vi "AOD.vi"() -> ()   [LabVIEW 2012]
uses:
  <vilib>/DAQmx/configure/timing.llb/DAQmx Timing (Sample Clock).vi
  <vilib>/DAQmx/configure/trigger.llb/DAQmx Start Trigger (Digital Edge).vi
  <resource>/objmgr/daqmx.rc
  <vilib>/DAQmx/configure/timing.llb/DAQmx Timing (Implicit).vi
  <vilib>/DAQmx/read.llb/DAQmx Read (Analog 1D Wfm NChan NSamp).vi
  <instrlib>/niHWS/nihws.llb/niHWS Open File Permissions ID.ctl
  <instrlib>/niHWS/nihws.llb/niHWS Write Analog WDT.vi
  <vilib>/DAQmx/read.llb/DAQmx Read (Digital 2D U32 NChan NSamp).vi
  <instrlib>/niHWS/nihws.llb/niHWS Write Digital 2D U32.vi
panel:
  in  "Channel":i32
  in  "Record":bool
  in  "Construct image":bool=TRUE
  in  "Show traces":bool
  in  "samples per ch":i32=5000
  out "PMT Waveforms":waveform(dbl)[](graph)
  out "Sync Signals":digitalwaveform(graph)
  out "Numeric":i32
  in  "stop":bool
  in  "buffer size":i32=10000000
  in  "pulse width (us)":dbl=5.0 format="%#.6f"
  in  "pixel oversampling":dbl=4.0
  in  "pixel rate":dbl=50000.0 format="%0.0f"
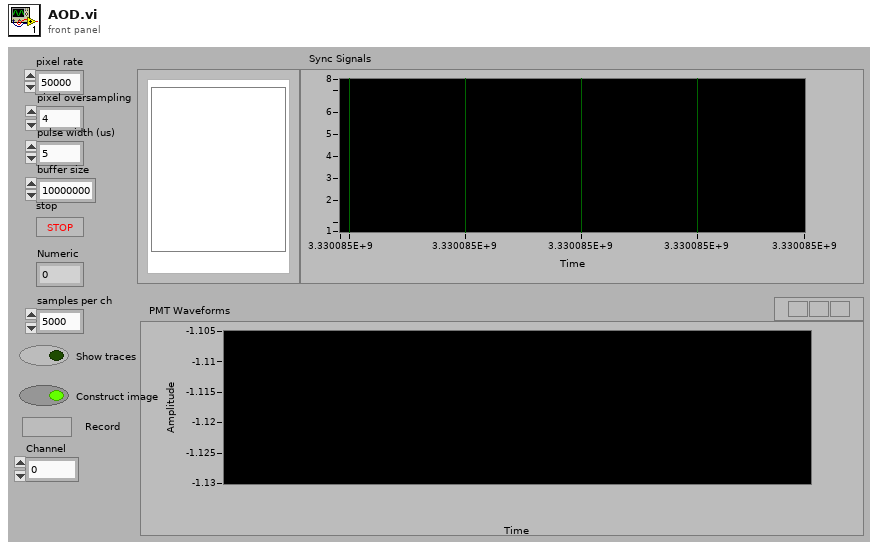
[diagram p1: front panel]
types:
  T1 = typedef "niHWS Open File Permissions ID.ctl" = enum32{"Read Only", "Read/Write Existing", "Read/Write/Create New", "Read/Write/Create New Always"}
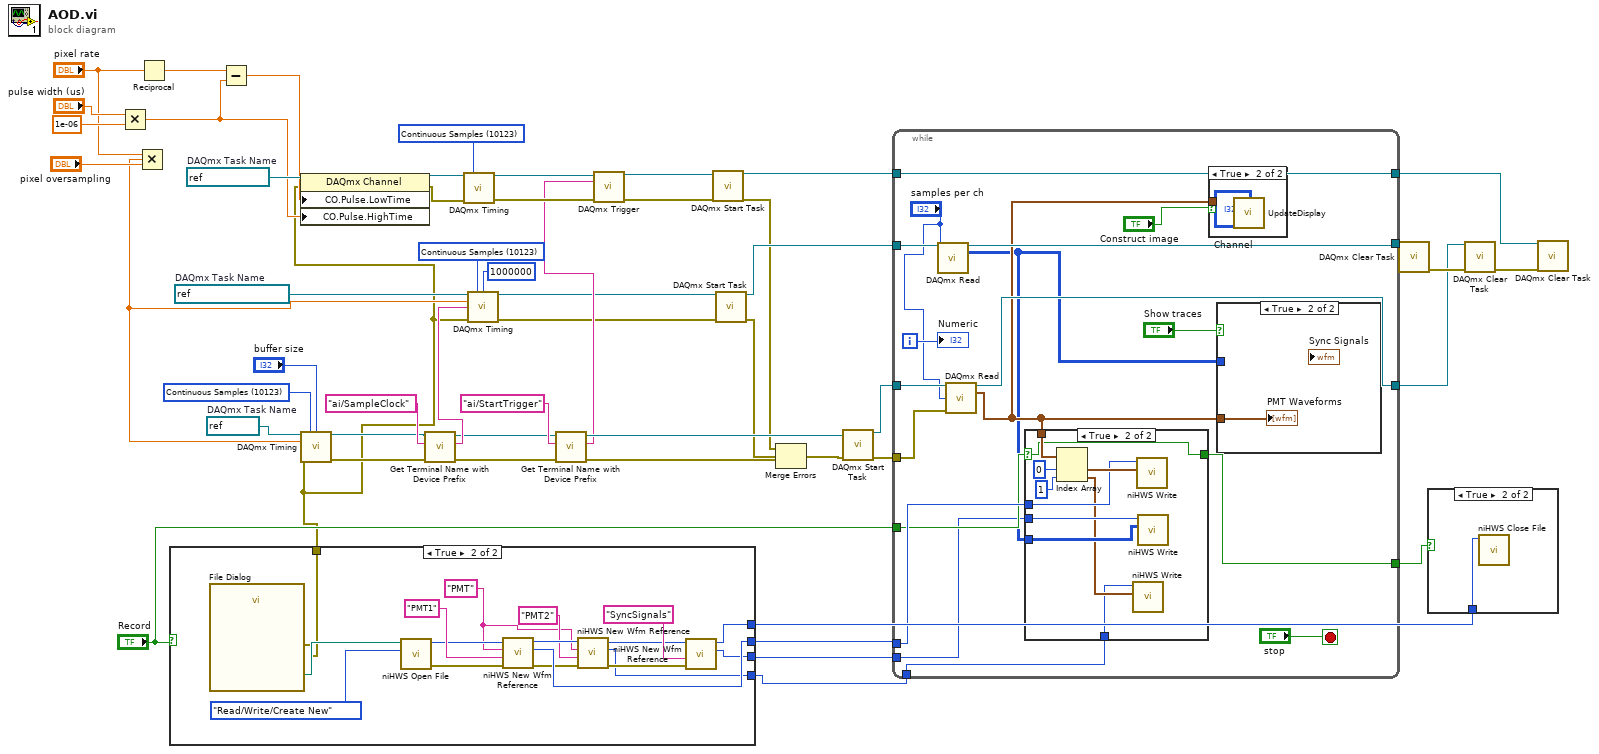
[diagram p0: block diagram]
diagram:
  w6 = 10123 items=["Finite Samples"=10178, "Continuous Samples"=10123, "Hardware Timed Single Point"=12522] ("sample mode")
  w36 = refnum<k21> "AODSyncSignals"  # DAQmx Task Name
  w42 = refnum<k21> "AODClock"  # DAQmx Task Name
  w47 = 10123 items=["Finite Samples"=10178, "Continuous Samples"=10123, "Hardware Timed Single Point"=12522] ("sample mode")
  w51 = refnum<k21> "PMT"  # DAQmx Task Name
  w53 = 10123 items=["Finite Samples"=10178, "Continuous Samples"=10123, "Hardware Timed Single Point"=12522] ("sample mode")
  n1 = Multiply(x="pulse width (us)", y=1e-06) -> (x*y=w37:dbl)
  n2 = Multiply(x="pixel rate", y="pixel oversampling") -> (x*y=w12:dbl)
  n3 = Reciprocal(x="pixel rate") -> (1/x=w39:dbl)
  n4 = case shown="True" "Record" {
    tunnel: [_ w67] -> w10
    tunnel: [_ w66] -> w8
    tunnel: [_ w63] -> w7
    tunnel: [_ w61] -> w2
    tunnel: [_ w54] -> w1
    frame False {
    }
    frame True {
      w55 = "PMT" ("group name (empty)")
      n5 = call "File Dialog"() -> ("selected path"=w62:path, "error out"=w61:errorcluster)  [unwired: 7 in, 7 out]
      n6 = call <instrlib>:"niHWS Open File.vi"("permissions (0:read only)"=niHWS_Open_File_Permissions_ID."Read/Write/Create New", "file path"=w62) -> ("error out"=w64:errorcluster, "file handle"=w68:u32)  [unwired: 1 in, 7 out]
      n7 = call <instrlib>:"niHWS New Wfm Reference.vi"("error in (no error)"=w64, "waveform name (empty)"="PMT1", "group name (empty)"=w55, "file handle in"=w68) -> ("error out"=w59:errorcluster, "waveform reference"=w67:u32, "file handle out"=w60:u32)  [unwired: 1 in, 4 out]
      n8 = call <instrlib>:"niHWS New Wfm Reference.vi"("error in (no error)"=w59, "waveform name (empty)"="PMT2", "group name (empty)"=w55, "file handle in"=w60) -> ("error out"=w58:errorcluster, "waveform reference"=w54:u32, "file handle out"=w57:u32)  [unwired: 1 in, 4 out]
      n9 = call <instrlib>:"niHWS New Wfm Reference.vi"("error in (no error)"=w58, "waveform name (empty)"="SyncSignals", "file handle in"=w57) -> ("waveform reference"=w63:u32, "file handle out"=w66:u32)  [unwired: 1 in, 6 out]
    }
  }
  n10 = Subtract(x=w39, y=w37) -> (x-y=w38:dbl)
  n11 = property class="DAQmx Channel"(reference=w42, error in=w2, "CO.Pulse.LowTime"=w38, "CO.Pulse.HighTime"=w37) -> (reference out=w40:refnum<k21>, error out=w41:errorcluster)
  n12 = call-poly <vilib>:"DAQmx Timing.vi"("task/channels in"=w51, "sample mode"=w47, "samples per channel"="buffer size", "rate"=w12, "error in"=w2) -> ("task out"=w30:refnum<k21>, "error out"=w35:errorcluster)  [unwired: 2 in, 7 out]
  n13 = call "Get Terminal Name with Device Prefix.vi"("error in (no error)"=w35, "Local Terminal Name"="ai/SampleClock", "task/channels in"=w30) -> ("error out"=w29:errorcluster, "Terminal Name with Device Prefix"=w33:tag, "task out"=w28:refnum<k21>)  [unwired: 1 in, 5 out]
  n14 = call-poly <vilib>:"DAQmx Timing.vi"("task/channels in"=w40, "sample mode"=w53, "error in"=w41) -> ("task out"=w46:refnum<k21>, "error out"=w45:errorcluster)  [unwired: 3 in, 8 out]
  n15 = call-poly <vilib>:"DAQmx Timing.vi"("task/channels in"=w36, "sample mode"=w6, "samples per channel"=1000000, "rate"=w12, "source"=w33, "error in"=w2) -> ("task out"=w4:refnum<k21>, "error out"=w3:errorcluster)  [unwired: 1 in, 7 out]
  n16 = call "Get Terminal Name with Device Prefix.vi"("error in (no error)"=w29, "Local Terminal Name"="ai/StartTrigger", "task/channels in"=w28) -> ("error out"=w27:errorcluster, "Terminal Name with Device Prefix"=w25:tag, "task out"=w26:refnum<k21>)  [unwired: 1 in, 5 out]
  n17 = call-poly <vilib>:"DAQmx Trigger.vi"("task/channels in"=w46, "source"=w25, "error in"=w45) -> ("task out"=w43:refnum<k21>, "error out"=w44:errorcluster)  [unwired: 1 in, 10 out]
  n18 = call <vilib>:"DAQmx Start Task.vi"("task/channels in"=w43, "error in"=w44) -> ("task out"=w22:refnum<k21>, "error out"=w17:errorcluster)  [unwired: 12 out]
  n19 = call <vilib>:"DAQmx Start Task.vi"("task/channels in"=w4, "error in"=w3) -> ("task out"=w24:refnum<k21>, "error out"=w16:errorcluster)  [unwired: 12 out]
  n20 = Merge Errors(w17, w16, w27) -> (w32:errorcluster)
  n21 = call <vilib>:"DAQmx Start Task.vi"("task/channels in"=w26, "error in"=w32) -> ("task out"=w19:refnum<k21>, "error out"=w18:errorcluster)  [unwired: 12 out]
  n22 = while {
    tunnel: w24 -> [w88]
    tunnel: [w86] -> w23
    tunnel: w22 -> [w81]
    tunnel: w19 -> [w84]
    tunnel: w18 -> [w83]
    tunnel: [w82] -> w15
    tunnel: [w81] -> w14
    tunnel: "Record" -> [w76]
    tunnel: w10 -> [w77]
    tunnel: [w74] -> w9
    tunnel: w7 -> [w73]
    tunnel: w1 -> [w71]
    i -> [w85]
    stop <- "stop" stop-if-true
    n23 = call-poly <vilib>:"DAQmx Read.vi"("task/channels in"=w88, "number of samples per channel"="samples per ch") -> ("task out"=w86:refnum<k21>, "data"=w72:u32[][])  [unwired: 1 in, 11 out]
    n24 = call-poly <vilib>:"DAQmx Read.vi"("task/channels in"=w84, "number of samples per channel"="samples per ch", "error in"=w83) -> ("task out"=w82:refnum<k21>, "data"=w75:waveform(dbl)[])  [unwired: 11 out]
    n25 = case shown="True" w76 {
      selector: w76 -> [w89 w95]
      tunnel: w75 -> [_ w99]
      tunnel: w77 -> [_ w96]
      tunnel: [w89 w95] -> w74
      tunnel: w73 -> [_ w94]
      tunnel: w72 -> [_ w93]
      tunnel: w71 -> [_ w90]
      frame False {
      }
      frame True {
        n26 = Index Array(array=w99, index #1=0 ("index"), index #2=1 ("index")) -> (element #1=w97:waveform(dbl), element #2=w91:waveform(dbl))
        n27 = call-poly <instrlib>:"niHWS Write.vi"("analog waveform"=w91, "waveform reference in"=w90) -> ()  [unwired: 1 in, 9 out]
        n28 = call-poly <instrlib>:"niHWS Write.vi"("analog waveform"=w97, "waveform reference in"=w96) -> ()  [unwired: 1 in, 9 out]
        n29 = call-poly <instrlib>:"niHWS Write.vi"("data"=w93, "waveform reference in"=w94) -> ()  [unwired: 1 in, 9 out]
      }
    }
    n30 = case shown="True" "Construct image" {
      tunnel: w75 -> [_ w101]
      frame False {
      }
      frame True {
        n31 = call "UpdateDisplay.vi"("Channel"="Channel", "Array"=w101) -> ()  [unwired: 10 out]
      }
    }
    n32 = case shown="True" "Show traces" {
      tunnel: w72 -> [_ _]
      tunnel: w75 -> [_ w102]
      frame False {
      }
      frame True {
        "PMT Waveforms" <- w102
      }
    }
    "Numeric" <- w85
  }
  n33 = call <vilib>:"DAQmx Clear Task.vi"("task in"=w23) -> ("error out"=w21:errorcluster)  [unwired: 1 in, 13 out]
  n34 = case shown="True" w9 {
    tunnel: w8 -> [_ w103]
    frame False {
    }
    frame True {
      n35 = call <instrlib>:"niHWS Close File.vi"("file handle"=w103) -> ()  [unwired: 1 in, 10 out]
    }
  }
  n36 = call <vilib>:"DAQmx Clear Task.vi"("task in"=w15, "error in"=w21) -> ("error out"=w20:errorcluster)  [unwired: 13 out]
  n37 = call <vilib>:"DAQmx Clear Task.vi"("task in"=w14, "error in"=w20) -> ()  [unwired: 14 out]
